vi "Epoch_NotationLocale.vi"(10 "custom":string, 11 "Delimiter (system)":T1) -> (3 "delimiter format":string)   [LabVIEW 2013]
uses:
  Locale -- enum.ctl
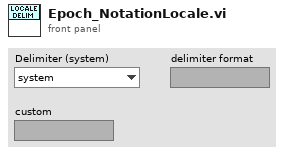
[diagram p1: front panel]
types:
  T1 = typedef "Locale -- enum.ctl" = enum16{"system", "Dot notation", "Comma notation", "custom"}
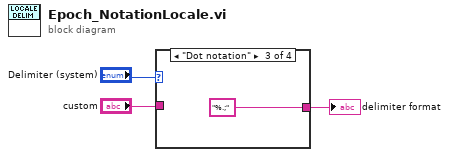
[diagram p0: block diagram]
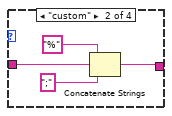
[diagram p3: hidden frame]
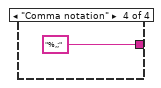
[diagram p4: hidden frame]
diagram:
  n1 = case shown="\"Dot notation\"" "Delimiter (system)" {
    tunnel: [_ w7 "%.;" "%,;"] -> w2
    tunnel: "custom" -> [_ w6 _ _]
    frame "system" {
    }
    frame "custom" {
      n2 = Concatenate Strings("%", w6, ";") -> (w7:string)
    }
    frame "Dot notation" {
    }
    frame "Comma notation" {
    }
  }
  "delimiter format" <- w2
